vi "Periodic Tasks.vi"(8 "error in":errorcluster, 11 "HARDWARE cluster":T1={"DRIVE MOTORS"=[], "Controller"=[], "ENCODERS"=[], "GYRO HARDWARE"={"Descr"="GYRO", "Installed?"=FALSE, "SPI Bus"=enum."SPI On-Board, CS0", "AnalogChannel"=enum."AI 0", "Calibrate On Open"=TRUE, "Calibrated Center Voltage"=0.0, "Calibration Time (s)"=2.0, "Sample Rate (Hz)"=100.0, "RefName"="", "stack name"="GYRO"}, "AIR"={"PRESSURE"=[], "COMPRESSOR"={"Descr"="COMPRESSOR", "Installed?"=TRUE, "Pneumatics Control Module"=0, "RefName"="COMPRESSOR", "stack name"="COMPRESSOR"}, "SOLENOIDS"=[]}, "MOTORS"=[], "SERVOS"=[], "SONAR"=[], "RELAY"=[], "LIMIT"=[]} {"MOTORS"."CAN ID" min=1 max=62 step=1; "MOTORS"."Motor Controller" items=["SPARK MAX", "SPARK", "Existing", "SD540", "TALON SRX", "VICTOR SP", "TALON SR", "JAGUAR", "VICTOR"]; "AIR"."PRESSURE"."warning HIGH" format="%.2f"; "AIR"."PRESSURE"."warning LOW" format="%.2f"; "AIR"."PRESSURE"."nominal value" format="%.2f"; "DRIVE MOTORS"."CAN ID" min=1 max=62 step=1; "DRIVE MOTORS"."Motor Controller" items=["SPARK MAX", "SPARK", "Existing", "SD540", "TALON SRX", "VICTOR SP", "TALON SR", "JAGUAR", "VICTOR"]; "Controller"."Parameters"."DEADBAND" format="%#_13g"; "Controller"."Parameters"."MIN SPEED" format="%#_13g"; "Controller"."Parameters"."MAX LIMIT" format="%#_13g"}) -> ()   [LabVIEW 2019]
doc: "This VI runs in parallel to other tasks. It can contain as many user-defined periodic loops as you need. These can carry out PID or other sorts of timed response."
uses:
  Controls/def HARDWARE CTRL info.ctl
  Controls/def MOTOR info.ctl
  Controls/ctrl MOTOR CTRLR SELECT.ctl
  <vilib>/Rock Robotics/SystemInterfaces/DIO/FPGA_DIOPWMChannel.ctl
  <vilib>/Rock Robotics/WPI/ThirdParty/REV Robotics/SPARK MAX/Typedef/Spark MAX Motor Type.ctl
  Controls/def USER CONTROL info.ctl
  <vilib>/Rock Robotics/WPI/Joystick/WPI_JoystickDeviceEnum.ctl
  Controls/def JOYSTICK PARAMETERS.ctl
  Controls/def ENCODER info.ctl
  <vilib>/Rock Robotics/SystemInterfaces/DIO/FPGA_DIOChannel.ctl
  <vilib>/Rock Robotics/WPI/Encoder/WPI_EncoderType.ctl
  Controls/def GYRO info.ctl
  <vilib>/Rock Robotics/SystemInterfaces/spilib/spi_bus.ctl
  Controls/ctrl ANALOG CHANNEL SELECT.ctl
  Controls/def AIR PRESSURE info.ctl
  <vilib>/Rock Robotics/SystemInterfaces/AI/FPGA_AIChannel.ctl
  Controls/def COMPRESSOR info.ctl
  Controls/def SOLENOID info.ctl
  <vilib>/Rock Robotics/WPI/Solenoid/WPI_SolenoidChannel.ctl
  <vilib>/Rock Robotics/WPI/Solenoid/WPI_SolenoidValue.ctl
  Controls/def SERVO info.ctl
  Controls/def SONAR info.ctl
  Controls/ctrl SONAR DEVICE SELECT.ctl
  <vilib>/Rock Robotics/WPI/Ultrasonic/WPI_UltrasonicRangeUnits.ctl
  Controls/def RELAY info.ctl
  <vilib>/Rock Robotics/SystemInterfaces/DIO/FPGA_DIORelayChannel.ctl
  <vilib>/Rock Robotics/WPI/Relay/WPI_RelayDirection.ctl
  <vilib>/Rock Robotics/WPI/Relay/WPI_RelayValue.ctl
  Controls/def LIMIT SWITCH info.ctl
  <vilib>/Rock Robotics/Network Tables/NT Write Number.vi
  Global  HARDWARE.vi
  <vilib>/Rock Robotics/Network Tables/NT Write Boolean.vi
  <vilib>/Rock Robotics/Network Tables/NT Read Boolean.vi
panel:
  in  "System loop time stack":string="/System/LOOPS/Periodic/start"
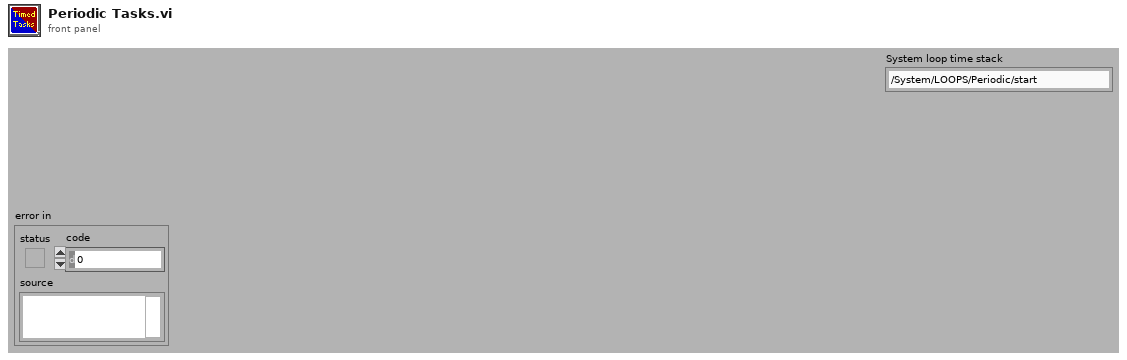
[diagram p1: front panel]
types:
  T1 = typedef "def HARDWARE CTRL info.ctl" = cluster{"DRIVE MOTORS":T2[], "Controller":T6[], "ENCODERS":T9[], "GYRO HARDWARE":T12, "AIR":cluster{"PRESSURE":T15[], "COMPRESSOR":T17, "SOLENOIDS":T18[]}, "MOTORS":T2[], "SERVOS":T21[], "SONAR":T22[], "RELAY":T25[], "LIMIT":T29[]}
  T2 = typedef "def MOTOR info.ctl" = cluster{"Descr":string, "Installed?":bool, "Protocol":enum16{"PWM", "CAN"}, "Motor Controller":T3, "PWM ch":T4, "RefName":string, "Invert?":bool, "stack name":string, "remove deadband":bool, "CAN ID":u8, "IDLE":string, "Motor Type":T5}
  T3 = typedef "ctrl MOTOR CTRLR SELECT.ctl" = u16
  T4 = typedef "FPGA_DIOPWMChannel.ctl" = enum8{"PWM 0", "PWM 1", "PWM 2", "PWM 3", "PWM 4", "PWM 5", "PWM 6", "PWM 7", "PWM 8", "PWM 9", "PWM MXP 0", "PWM MXP 1", "PWM MXP 2", "PWM MXP 3", "PWM MXP 4", "PWM MXP 5", "PWM MXP 6", "PWM MXP 7", "PWM MXP 8", "PWM MXP 9", "Invalid"}
  T5 = typedef "Spark MAX Motor Type.ctl" = enum16{"Brushed", "Brushless"}
  T6 = typedef "def USER CONTROL info.ctl" = cluster{"Descr":string, "Installed?":bool, "RefName":string, "JoystickDevice":T7, "Invert Y axis":bool, "Scale":dbl, "AXIS":string, "BUTTONS":string, "POV":string, "Parameters":T8}
  T7 = typedef "WPI_JoystickDeviceEnum.ctl" = enum16{"USB 0", "USB 1", "USB 2", "USB 3", "USB 4", "USB 5"}
  T8 = typedef "def JOYSTICK PARAMETERS.ctl" = cluster{"MAX LIMIT":dbl, "MIN SPEED":dbl, "DEADBAND":dbl, "invert X?":bool, "invert Y?":bool}
  T9 = typedef "def ENCODER info.ctl" = cluster{"Descr":string, "Installed?":bool, "A Channel":T10, "B Channel":T10, "Invert Direction":bool, "Enum":T11, "Gear ratio":dbl, "Cycles per Rev":dbl, "Diameter (in)":dbl[unit], "RefName":string, "stack name":string, "min rate (hz)":dbl, "Samples":u8, "STACK subnames":cluster{"RESET name":string, "STOPPED name":string, "DIRECTION name":string, "RATE name":string, "INSTALLED name":string}}
  T10 = typedef "FPGA_DIOChannel.ctl" = enum8{"DIO 0", "DIO 1", "DIO 2", "DIO 3", "DIO 4", "DIO 5", "DIO 6", "DIO 7", "DIO 8", "DIO 9", "DIO MXP 0", "DIO MXP 1", "DIO MXP 2", "DIO MXP 3", "DIO MXP 4", "DIO MXP 5", "DIO MXP 6", "DIO MXP 7", "DIO MXP 8", "DIO MXP 9", "DIO MXP 10", "DIO MXP 11", "DIO MXP 12", "DIO MXP 13", "DIO MXP 14", "DIO MXP 15", "SPI Port CS1", "SPI Port CS2", "SPI Port CS3", "SPI Port MISO", "SPI Port MOSI", "Invalid"}
  T11 = typedef "WPI_EncoderType.ctl" = enum16{"1x", "2x", "4x"}
  T12 = typedef "def GYRO info.ctl" = cluster{"Descr":string, "Installed?":bool, "SPI Bus":T13, "AnalogChannel":T14, "Calibrate On Open":bool, "Calibrated Center Voltage":dbl, "Calibration Time (s)":dbl, "Sample Rate (Hz)":dbl, "RefName":string, "stack name":string}
  T13 = typedef "spi_bus.ctl" = enum16{"SPI On-Board, CS0", "SPI On-Board, CS1", "SPI On-Board, CS2", "SPI On-Board, CS3", "SPI MXP", "Invalid"}
  T14 = typedef "ctrl ANALOG CHANNEL SELECT.ctl" = enum8{"AI 0", "AI 1", "Invalid"}
  T15 = typedef "def AIR PRESSURE info.ctl" = cluster{"Descr":string, "Installed?":bool, "Channel":T16, "RefName":string, "stack name":string, "MULTIPLIER":dbl, "OFFSET":dbl, "nominal value":dbl, "warning LOW":dbl, "warning HIGH":dbl}
  T16 = typedef "FPGA_AIChannel.ctl" = enum8{"AI 0", "AI 1", "AI 2", "AI 3", "AI MXP 0", "AI MXP 1", "AI MXP 2", "AI MXP 3", "Invalid"}
  T17 = typedef "def COMPRESSOR info.ctl" = cluster{"Descr":string, "Installed?":bool, "Pneumatics Control Module":u8, "RefName":string, "stack name":string}
  T18 = typedef "def SOLENOID info.ctl" = cluster{"Descr":string, "Installed?":bool, "Pneumatics Control Module (0)":u8, "DBL":bool, "SolenoidChannel":T19, "SolenoidChannel":T19, "Default SET":T20, "RefName":string, "Value":string}
  T19 = typedef "WPI_SolenoidChannel.ctl" = enum8{"Solenoid 0", "Solenoid 1", "Solenoid 2", "Solenoid 3", "Solenoid 4", "Solenoid 5", "Solenoid 6", "Solenoid 7", "Invalid"}
  T20 = typedef "WPI_SolenoidValue.ctl" = enum16{"Off", "On", "Forward", "Reverse"}
  T21 = typedef "def SERVO info.ctl" = cluster{"Descr":string, "PWM ch":T4, "Installed?":bool, "Angular range":dbl, "RefName":string, "stack name":string}
  T22 = typedef "def SONAR info.ctl" = cluster{"Descr":string, "Installed?":bool, "Device type":T23, "PING Channel":T10, "ECHO Channel":T10, "RefName":string, "stack name":string, "Samples":i32, "Range Units":T24}
  T23 = typedef "ctrl SONAR DEVICE SELECT.ctl" = enum16{"SRF04 Digital", "MB1010 Digital", "MB1010 Analog", "SRF08 Digital"}
  T24 = typedef "WPI_UltrasonicRangeUnits.ctl" = enum16{"inches", "mm"}
  T25 = typedef "def RELAY info.ctl" = cluster{"Descr":string, "Installed?":bool, "RelayChannel":T26, "Relay Direction":T27, "Relay Value":T28, "RefName":string, "Value":string}
  T26 = typedef "FPGA_DIORelayChannel.ctl" = enum8{"Relay 0", "Relay 1", "Relay 2", "Relay 3", "Invalid"}
  T27 = typedef "WPI_RelayDirection.ctl" = enum16{"Both directions", "Forward only", "Reverse only"}
  T28 = typedef "WPI_RelayValue.ctl" = enum16{"Off", "On", "Forward", "Reverse"}
  T29 = typedef "def LIMIT SWITCH info.ctl" = cluster{"Descr":string, "Installed?":bool, "A Channel":T10, "Normally Closed?":bool, "RefName":string, "stack name":string}
  T30 = typedef "ctrl LOOP TIMES def.ctl" = cluster{"Input controllers":u8, "Drive system":u8, "Encoders":u8, "Limit switches":u8, "Sonar":u8, "Servos":u8, "Gyro":u8, "AIR PRESS":u8, "Solenoids":u8, "Motors":u8}
  T31 = typedef "WPI_JoystickDevRef.ctl" = cluster{"Device":T7}
  T32 = typedef "WPI_EncoderDevRef.ctl" = cluster{"DevStatus":errorcluster, "EncoderIndex":T33, "CounterIndex":T34, "DistancePerCount":dbl, "Decoding Type":T11}
  T33 = typedef "FPGA_EncoderIdx.ctl" = enum8{"Enc 0", "Enc 1", "Enc 2", "Enc 3", "Enc 4", "Enc 5", "Enc 6", "Enc 7", "Invalid"}
  T34 = typedef "FPGA_CounterCtrSystemIndex.ctl" = enum8{"Ctr 0", "Ctr 1", "Ctr 2", "Ctr 3", "Ctr 4", "Ctr 5", "Ctr 6", "Ctr 7", "Invalid"}
  T35 = typedef "WPI_UltrasonicDeviceRef.ctl" = cluster{"DevStatus":errorcluster, "Ping Channel":T10, "Echo Channel":T10, "CntIndex":T34}
  T36 = typedef "WPI_SwitchDevRef.ctl" = cluster{"DevStatus":errorcluster, "DIO Channel":T10, "CntIndex":T34, "Normally Closed":bool}
  T37 = typedef "WPI_AnalogChannelDevRef.ctl" = cluster{"DevStatus":errorcluster, "Analog Channel":T16}
  T38 = typedef "WPI_RobotDriveDevRef.ctl" = cluster{"DevStatus":errorcluster, "Motors[]":T39[], "Square Inputs":bool, "Max Output":dbl}
  T39 = typedef "WPI_MotorControlDeviceRef.ctl" = cluster{"DeviceStatus":errorcluster, "Type":T40, "PWM":cluster{"PWM Channel":T4, "DeadBand":T41}, "CAN":cluster{"Device Number":u8, "SetOutput VI Ref":variant, "GetOutput VI Ref":variant, "Enable VI Ref":variant, "Disable VI Ref":variant, "Data":variant}, "Invert":bool, "DIO PWM":cluster{"PWM \"Enable\" Channel":T4, "DIOChannel":T10, "PWM Rate":dbl}}
  T40 = typedef "WPI_MotorControlType.ctl" = enum16{"PWM", "CAN", "DIO PWM"}
  T41 = typedef "WPI_PWMDeadband.ctl" = cluster{"Name":string, "maxPositivePwm":i32, "minPositivePwm":i32, "centerPwm":i32, "maxNegativePwm":i32, "minNegativePwm":i32, "angularRange":u16}
  T42 = cluster{"JoystickDevRef":T31, "RobotDriveDevRef":T38}
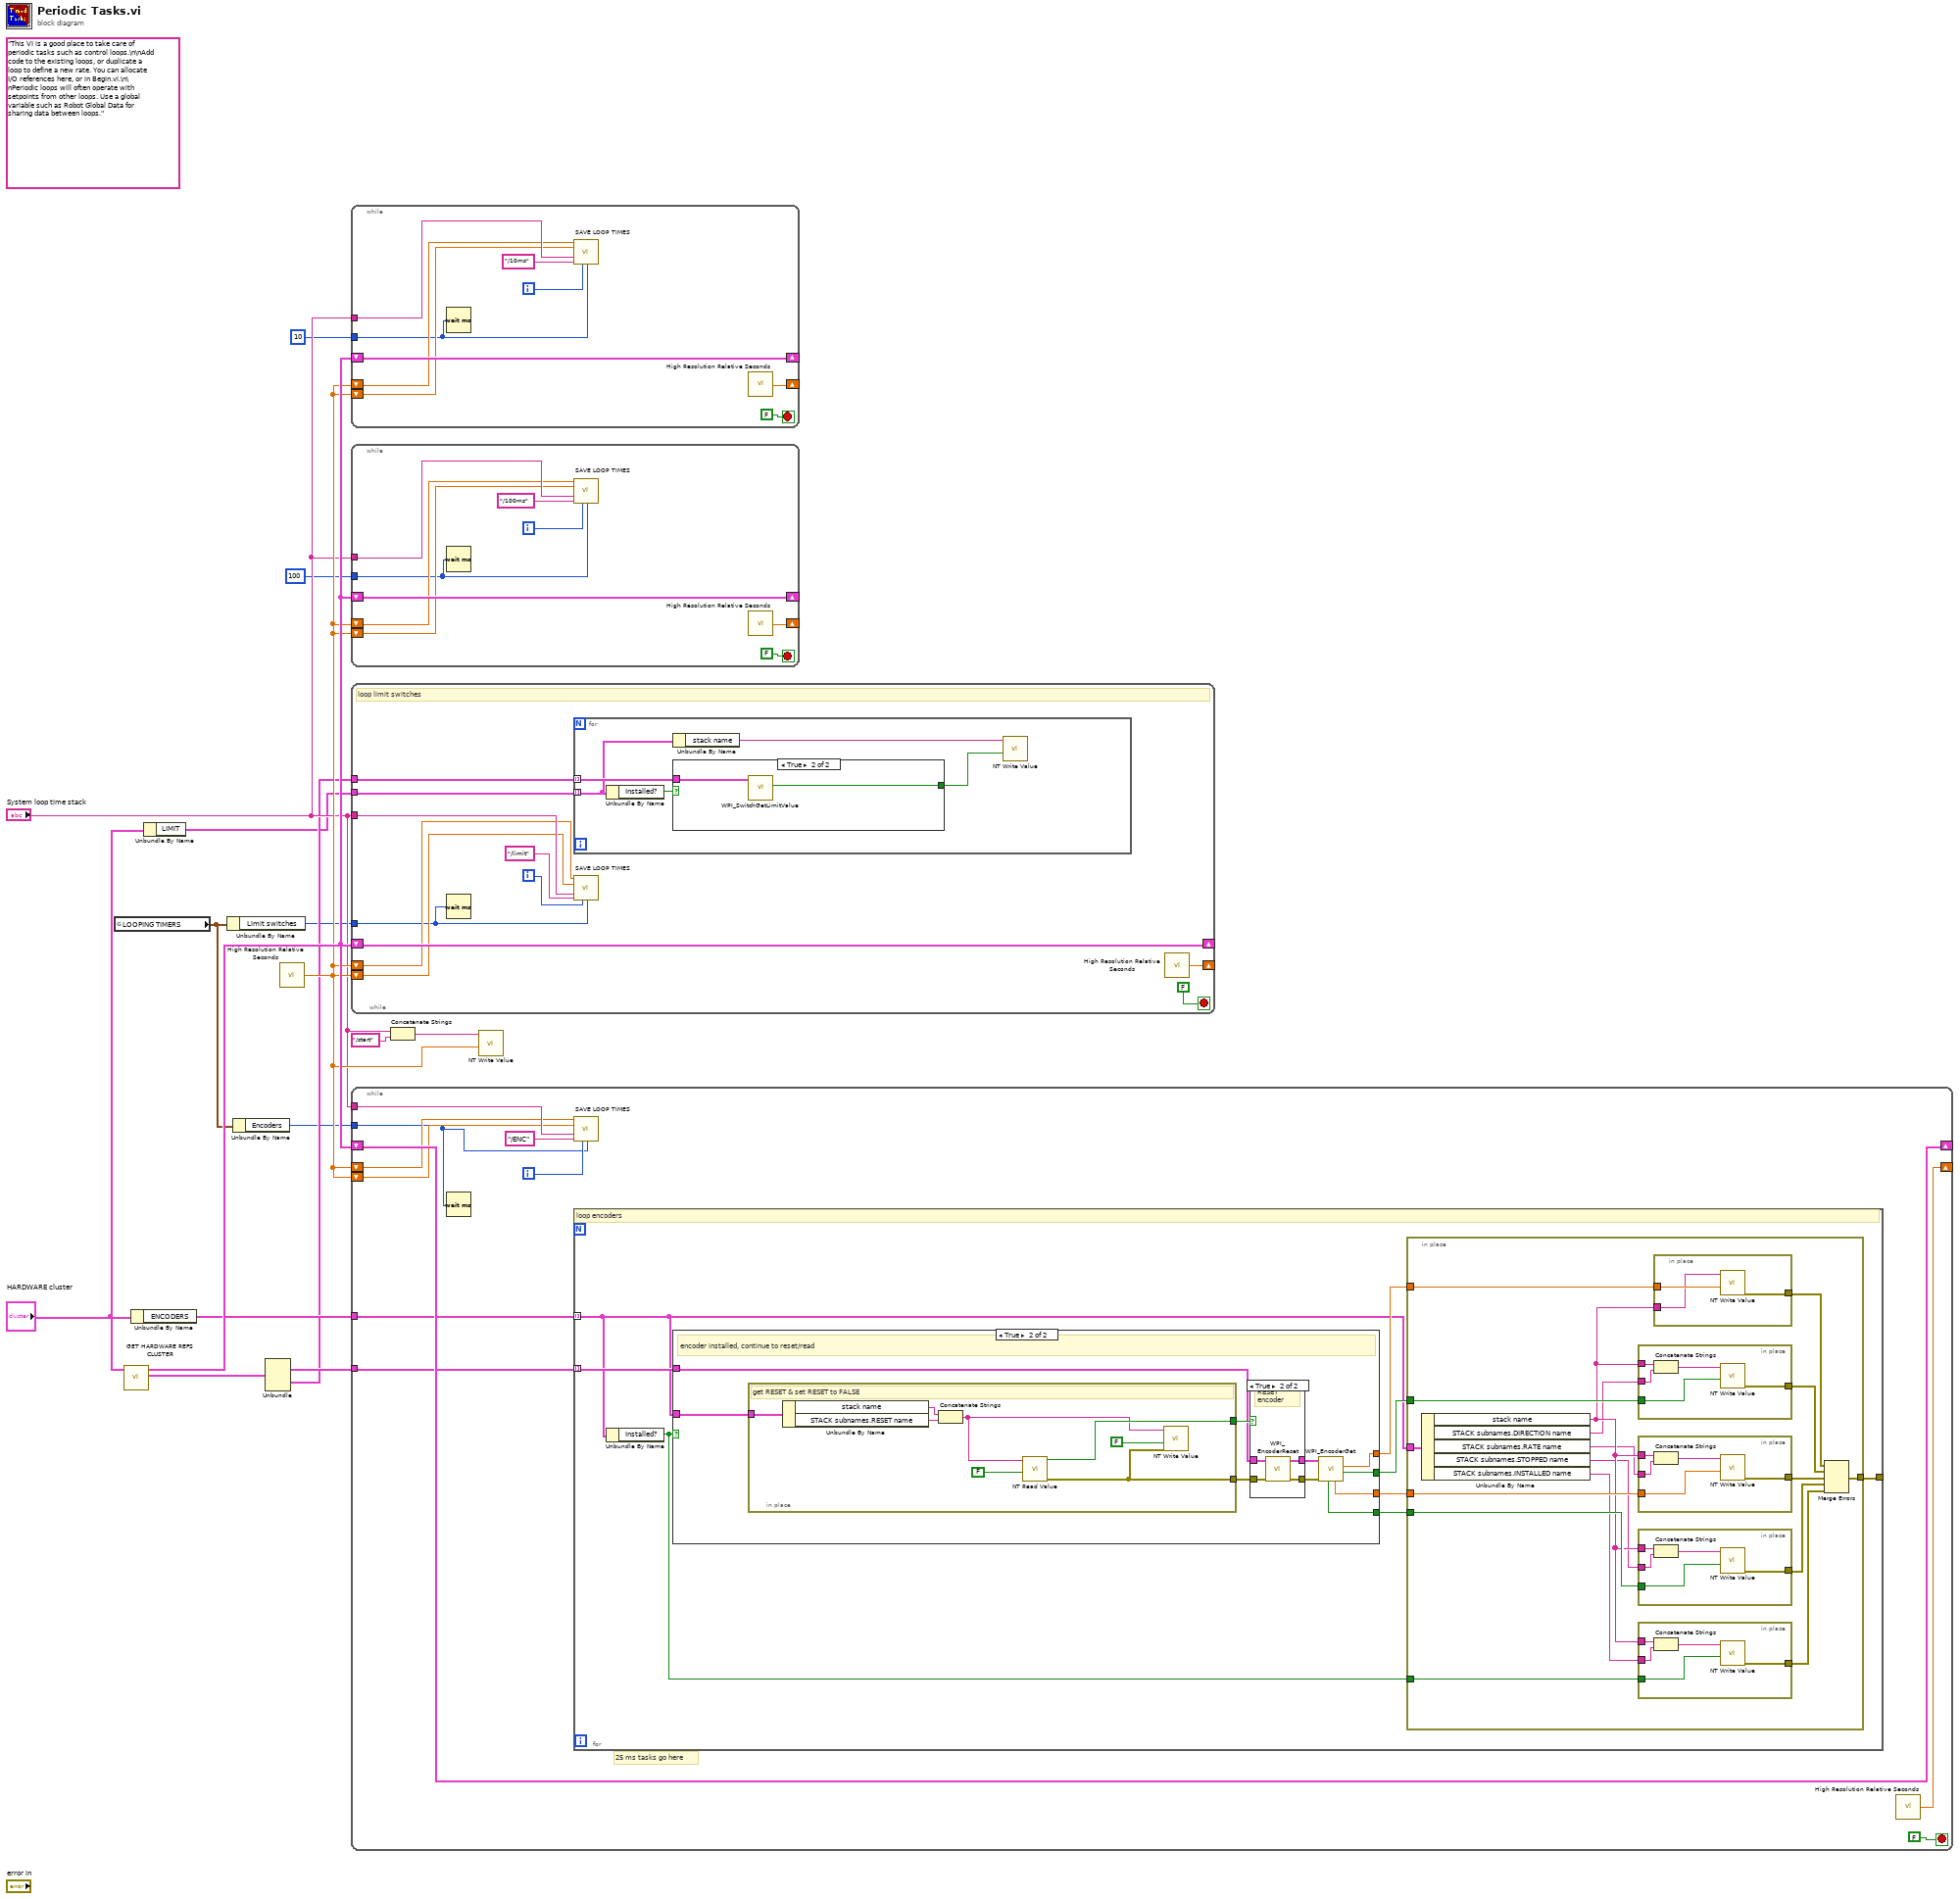
[diagram p0: block diagram]
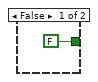
[diagram p2: hidden frame]
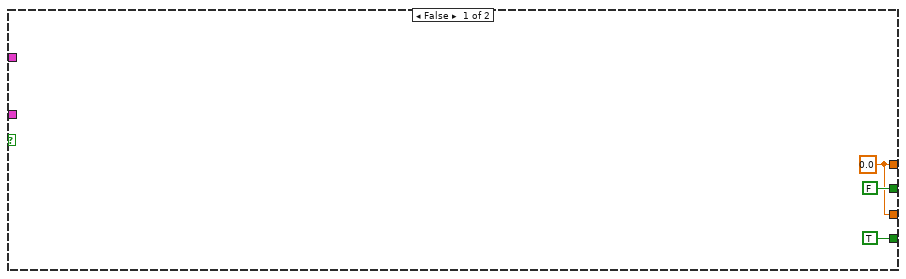
[diagram p3: hidden frame]
diagram:
  (unwired) "This VI is a good place to take care of periodic tasks such as control loops.\n\nAdd code to the existing loops, or duplicate a loop to define a new rate. You can allocate I/O references here, or in Begin.vi.\n\nPeriodic loops will often operate with setpoints from other loops. Use a global variable such as Robot Global Data for sharing data between loops."
  n1 = global read "Global  HARDWARE.vi" "LOOPING TIMERS"() -> (w2:T30)
  n2 = call "GET HARDWARE REFS CLUSTER.vi"("HARDWARE cluster"="HARDWARE cluster") -> ("REF INPUT"=w14:cluster{T31[], T32[], T35[], T36[], T37[]}, "REF DRIVE JOYSTICK"=w16:T42)  [unwired: 8 in, 1 out]
  n3 = Unbundle By Name("HARDWARE cluster") -> ("ENCODERS"=w15:T9[])
  n4 = Unbundle By Name("HARDWARE cluster") -> ("LIMIT"=w4:T29[])
  n5 = Unbundle By Name(w2) -> ("Limit switches"=w1:u8)
  n6 = Unbundle By Name(w2) -> ("Encoders"=w3:u8)
  n7 = Unbundle(w14) -> (w13:T32[], w6:T36[])  [unwired: 3 out]
  n8 = call <vilib>:"High Resolution Relative Seconds.vi"() -> ("relative seconds"=w10:dbl)
  n9 = while {
    shift-right: [w24] -> _
    shift-left: w16 -> [w24]
    tunnel: "System loop time stack" -> [w21]
    shift-right: [w23] -> _
    shift-left: w10 -> [w19]
    shift-left: w10 -> [w20]
    tunnel: u32 10 ("milliseconds to wait") -> [w17]
    i -> [w18]
    stop <- FALSE stop-if-true
    n10 = Wait (ms)(milliseconds to wait=w17) -> ()  [unwired: 1 out]
    n11 = call "SAVE LOOP TIMES.vi"("time this loop"=w19, "time last loop"=w20, "System loop time stack"=w21, "LOOP NAME"="/10ms" ("string"), "loop iteration"=w18, "milliseconds to wait"=w17) -> ()  [unwired: 9 in, 1 out]
    n12 = call <vilib>:"High Resolution Relative Seconds.vi"() -> ("relative seconds"=w23:dbl)
  }
  n13 = while {
    shift-right: [w33] -> _
    shift-left: w16 -> [w33]
    shift-right: [w32] -> _
    shift-left: w10 -> [w28]
    shift-left: w10 -> [w29]
    tunnel: "System loop time stack" -> [w30]
    tunnel: u32 100 ("milliseconds to wait") -> [w26]
    i -> [w27]
    stop <- FALSE stop-if-true
    n14 = Wait (ms)(milliseconds to wait=w26) -> ()  [unwired: 1 out]
    n15 = call "SAVE LOOP TIMES.vi"("time this loop"=w28, "time last loop"=w29, "System loop time stack"=w30, "LOOP NAME"="/100ms" ("string"), "loop iteration"=w27, "milliseconds to wait"=w26) -> ()  [unwired: 9 in, 1 out]
    n16 = call <vilib>:"High Resolution Relative Seconds.vi"() -> ("relative seconds"=w32:dbl)
  }
  n17 = while {
    shift-right: [w44] -> _
    shift-left: w16 -> [w44]
    shift-right: [w43] -> _
    shift-left: w10 -> [w39]
    shift-left: w10 -> [w40]
    tunnel: "System loop time stack" -> [w41]
    tunnel: w1 -> [w37]
    tunnel: w6 -> [w36]
    tunnel: w4 -> [w35]
    i -> [w38]
    stop <- FALSE stop-if-true
    # "loop limit switches"
    n18 = Wait (ms)(milliseconds to wait=w37) -> ()  [unwired: 1 out]
    n19 = for {
      tunnel: w36 -> [w49] mode=indexing
      tunnel: w35 -> [w48] mode=indexing
      n20 = Unbundle By Name(w48) -> ("Installed?"=w50:bool)
      n21 = Unbundle By Name(w48) -> ("stack name"=w47:string)
      n22 = case shown="True" w50 {
        tunnel: w49 -> [_ w53]
        tunnel: [FALSE ("Switch Pressed") w52] -> w46
        frame False {
        }
        frame True {
          n23 = call <vilib>:"WPI_SwitchGetLimitValue.vi"("SwitchDevRef"=w53) -> ("Switch Pressed"=w52:bool)  [unwired: 8 in, 2 out]
        }
      }
      n24 = call-poly <vilib>:"NT Write Value.vi"("Boolean"=w46, "Name"=w47) -> ()  [unwired: 9 in, 1 out]
    }
    n25 = call "SAVE LOOP TIMES.vi"("time this loop"=w39, "time last loop"=w40, "System loop time stack"=w41, "LOOP NAME"="/limit" ("string"), "loop iteration"=w38, "milliseconds to wait"=w37) -> ()  [unwired: 9 in, 1 out]
    n26 = call <vilib>:"High Resolution Relative Seconds.vi"() -> ("relative seconds"=w43:dbl)
  }
  n27 = while {
    shift-right: [w63] -> _
    shift-left: w16 -> [w63]
    tunnel: w15 -> [w62]
    tunnel: w13 -> [w61]
    shift-right: [w58] -> _
    shift-left: w10 -> [w57]
    tunnel: "System loop time stack" -> [w59]
    shift-left: w10 -> [w56]
    tunnel: w3 -> [w54]
    i -> [w55]
    stop <- FALSE stop-if-true
    # "25 ms tasks go here"
    n28 = Wait (ms)(milliseconds to wait=w54) -> ()  [unwired: 1 out]
    n29 = call "SAVE LOOP TIMES.vi"("time this loop"=w57, "time last loop"=w56, "System loop time stack"=w59, "LOOP NAME"="/ENC" ("string"), "loop iteration"=w55, "milliseconds to wait"=w54) -> ()  [unwired: 9 in, 1 out]
    n30 = for {
      tunnel: w62 -> [w65] mode=indexing
      tunnel: w61 -> [w68] mode=indexing
      tunnel: [w67] -> _
      # "loop encoders"
      n31 = Unbundle By Name(w65) -> ("Installed?"=w66:bool)
      n32 = case shown="True" w66 {
        tunnel: w68 -> [_ w124]
        tunnel: [w113 w122] -> w72
        tunnel: [FALSE ("Direction") w121] -> w71
        tunnel: [w113 w120] -> w70
        tunnel: [TRUE ("Stopped") w119] -> w69
        tunnel: w65 -> [_ w116]
        frame False {
          w113 = 0.0 ("Rate")
        }
        frame True {
          # "encoder installed, continue to reset/read"
          n33 = in-place {
            in-place-border: [w133] -> w125
            in-place-border: [w130] -> w118
            in-place-border: w116 -> [w128]
            # "get RESET & set RESET to FALSE"
            n34 = Unbundle By Name(w128) -> ("stack name"=w127:string, "STACK subnames.RESET name"=w126:string)
            n35 = Concatenate Strings(w127, w126) -> (w132:string)
            n36 = call-poly <vilib>:"NT Read Value.vi"("Default Value"=FALSE, "Name"=w132) -> ("error out"=w130:errorcluster, "Boolean"=w133:bool)  [unwired: 8 in]
            n37 = call-poly <vilib>:"NT Write Value.vi"("error in"=w130, "Boolean"=FALSE, "Name"=w132) -> ()  [unwired: 8 in, 1 out]
          }
          n38 = case shown="True" w125 {
            tunnel: w124 -> [w135 w139]
            tunnel: [w135 w138] -> w123
            tunnel: [w134 w137] -> w117
            tunnel: w118 -> [w134 w136]
            frame False {
            }
            frame True {
              # "RESET encoder"
              n39 = call <vilib>:"WPI_EncoderReset.vi"("error in (no error)"=w136, "EncoderDevRef"=w139) -> ("error out"=w137:errorcluster, "EncoderDevRef"=w138:T32)  [unwired: 8 in]
            }
          }
          n40 = call <vilib>:"WPI_EncoderGet.vi"("error in (no error)"=w117, "EncoderDevRef"=w123) -> ("Direction"=w121:bool, "Distance"=w122:dbl, "Rate"=w120:dbl, "Stopped"=w119:bool)  [unwired: 4 in, 2 out]
        }
      }
      n41 = in-place {
        in-place-border: w72 -> [w89]
        in-place-border: w71 -> [w88]
        in-place-border: w70 -> [w87]
        in-place-border: w69 -> [w86]
        in-place-border: [w85] -> w67
        in-place-border: w66 -> [w79]
        in-place-border: w65 -> [w78]
        n42 = Unbundle By Name(w78) -> ("stack name"=w77:string, "STACK subnames.DIRECTION name"=w76:string, "STACK subnames.RATE name"=w75:string, "STACK subnames.STOPPED name"=w74:string, "STACK subnames.INSTALLED name"=w73:string)
        n43 = in-place {
          in-place-border: w88 -> [w109]
          in-place-border: w77 -> [w108]
          in-place-border: [w106] -> w83
          in-place-border: w76 -> [w105]
          n44 = Concatenate Strings(w108, w105) -> (w107:string)
          n45 = call-poly <vilib>:"NT Write Value.vi"("Boolean"=w109, "Name"=w107) -> ("error out"=w106:errorcluster)  [unwired: 9 in]
        }
        n46 = in-place {
          in-place-border: w87 -> [w104]
          in-place-border: w77 -> [w103]
          in-place-border: [w101] -> w82
          in-place-border: w75 -> [w100]
          n47 = Concatenate Strings(w103, w100) -> (w102:string)
          n48 = call-poly <vilib>:"NT Write Value.vi"("Numeric"=w104, "Name"=w102) -> ("error out"=w101:errorcluster)  [unwired: 9 in]
        }
        n49 = in-place {
          in-place-border: w86 -> [w99]
          in-place-border: w77 -> [w98]
          in-place-border: [w96] -> w81
          in-place-border: w74 -> [w95]
          n50 = Concatenate Strings(w98, w95) -> (w97:string)
          n51 = call-poly <vilib>:"NT Write Value.vi"("Boolean"=w99, "Name"=w97) -> ("error out"=w96:errorcluster)  [unwired: 9 in]
        }
        n52 = in-place {
          in-place-border: w79 -> [w94]
          in-place-border: w77 -> [w93]
          in-place-border: [w91] -> w80
          in-place-border: w73 -> [w90]
          n53 = Concatenate Strings(w93, w90) -> (w92:string)
          n54 = call-poly <vilib>:"NT Write Value.vi"("Boolean"=w94, "Name"=w92) -> ("error out"=w91:errorcluster)  [unwired: 9 in]
        }
        n55 = in-place {
          in-place-border: w89 -> [w112]
          in-place-border: w77 -> [w111]
          in-place-border: [w110] -> w84
          n56 = call-poly <vilib>:"NT Write Value.vi"("Numeric"=w112, "Name"=w111) -> ("error out"=w110:errorcluster)  [unwired: 9 in]
        }
        n57 = Merge Errors(w84, w83, w82, w81, w80) -> (w85:errorcluster)
      }
    }
    n58 = call <vilib>:"High Resolution Relative Seconds.vi"() -> ("relative seconds"=w58:dbl)
  }
  n59 = Concatenate Strings("System loop time stack", "/start" ("string")) -> (w12:string)
  n60 = call-poly <vilib>:"NT Write Value.vi"("Numeric"=w10, "Name"=w12) -> ()  [unwired: 9 in, 1 out]
